vi "Array to VCluster__ogtk.vi"(8 "error in (no error)":errorcluster, 10 "Array":variant) -> (0 "error out":errorcluster, 2 "VCluster":variant)   [LabVIEW 2017]
doc: "Returns the elements of an array as elements of a variant cluster."
panel:
  # "[OpenG VI Tags] ***Do Not Remove***"
  # "Array to VCluster.vi\n\nReturns the elements of an array as elements of a variant cluster.\n\nPlease visit http://www.OpenG.org to learn about the\nOpen Source LabVIEW software movement.\n\nNOTICE -- YOU MUST LEAVE THIS NOTICE IN PLACE.  PER THE TERMS OF THE LICENSE BELOW, YOU MAY SUBLICENSE THIS SOFTWARE \nIN ANY WAY THAT DOES NOT CONFLICT WITH THIS LICENSE.\n\n### BSD License (http://www.opensource.org/licenses/bsd-license.php) Begin ###\n \nCopyright (c) 2002, Jean-Pierre Drolet <drolet_jp@hotmail.com>\nCopyright (c) 2002-2006, Jim Kring <jim@jimkring.com>\n\nAll rights reserved.\n\nRedistribution and use in source and binary forms, with or without modification, are permitted provided that the following conditions are met:\n\n    * Redistributions of source code must retain the above copyright notice, this list of conditions and the following disclaimer.\n    * Redistributions in binary form must reproduce the above copyright notice, this list of conditions and the following disclaimer in the \n       documentation and/or other materials provided with the distribution.\n    * Neither the name of SciWare, James Kring, Inc., nor the names of its contributors may be used to endorse or promote products derived \n       from this software without specific prior written permission.\n\nTHIS SOFTWARE IS PROVIDED BY THE COPYRIGHT HOLDERS AND CONTRIBUTORS \"AS IS\" AND ANY EXPRESS OR IMPLIED WARRANTIES, \nINCLUDING, BUT NOT LIMITED TO, THE IMPLIED WARRANTIES OF MERCHANTABILITY AND FITNESS FOR A PARTICULAR PURPOSE ARE \nDISCLAIMED. IN NO EVENT SHALL THE COPYRIGHT OWNER OR CONTRIBUTORS BE LIABLE FOR ANY DIRECT, INDIRECT, INCIDENTAL,\n SPECIAL, EXEMPLARY, OR CONSEQUENTIAL DAMAGES (INCLUDING, BUT NOT LIMITED TO, PROCUREMENT OF SUBSTITUTE GOODS OR \nSERVICES; LOSS OF USE, DATA, OR PROFITS; OR BUSINESS INTERRUPTION) HOWEVER CAUSED AND ON ANY THEORY OF LIABILITY, \nWHETHER IN CONTRACT, STRICT LIABILITY, OR TORT (INCLUDING NEGLIGENCE OR OTHERWISE) ARISING IN ANY WAY OUT OF THE USE \nOF THIS SOFTWARE, EVEN IF ADVISED OF THE POSSIBILITY OF SUCH DAMAGE.\n\n### BSD License End ###"
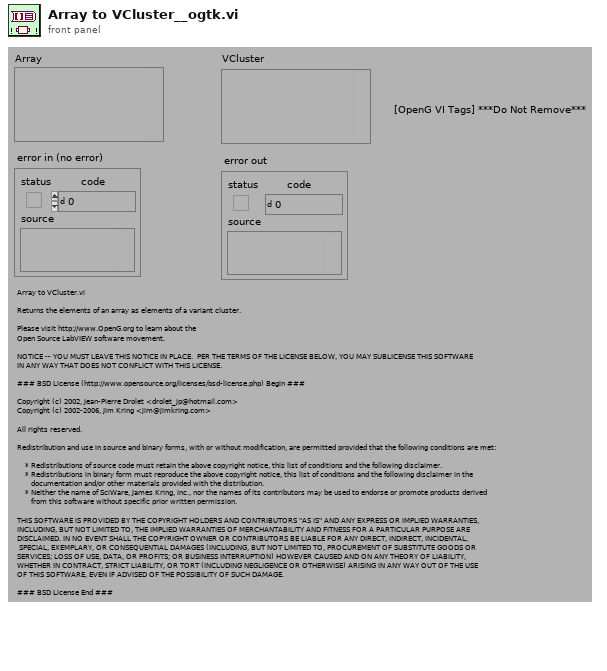
[diagram p1: front panel]
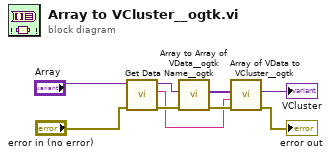
[diagram p0: block diagram]
diagram:
  n1 = call "Get Data Name__ogtk.vi"("error in (no error)"="error in (no error)", "Data"="Array") -> ("error out"=w5:errorcluster, "Data Name"=w1:string, "Data dup"=w3:variant)  [unwired: 7 in]
  n2 = call "Array to Array of VData__ogtk.vi"("error in (no error)"=w5, "MultiD Array"=w3) -> ("error out"=w8:errorcluster, "1D Array of Variants"=w9:variant[])  [unwired: 8 in]
  n3 = call "Array of VData to VCluster__ogtk.vi"("error in (no error)"=w8, "Cluster Name"=w1, "Array"=w9) -> ("error out"=→"error out":errorcluster, "VCluster"=→"VCluster":variant)  [unwired: 7 in]
